vi "LocalOrGlobalMeasurement.vi"(6 "Use Offsets":T1, 7 "Tag":string, 8 "Combined":bool, 9 "IsCommand":bool, 11 "Target":T2) -> (3 "Adjusted Target":T2)   [LabVIEW 2013]
uses:
  MixedMode/Messages/Target.ctl
  Data Access Objects/Metadata/LBCB Number.ctl
  Apps/On Off Button.ctl
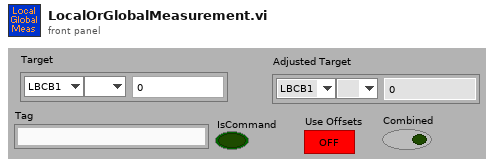
[diagram p1: front panel]
types:
  T1 = typedef "On Off Button.ctl" = bool
  T2 = typedef "Target.ctl" = cluster{"LBCB Number":T3, "DOF Vectors":enum16{" ", "Dx", "Dy", "Dz", "Rx", "Ry", "Rz", "Fx", "Fy", "Fz", "Mx", "My", "Mz"}, "Amount":dbl}
  T3 = typedef "LBCB Number.ctl" = enum16{"LBCB1", "LBCB2"}
  T4 = enum16{" ", "Dx", "Dy", "Dz", "Rx", "Ry", "Rz", "Fx", "Fy", "Fz", "Mx", "My", "Mz"}
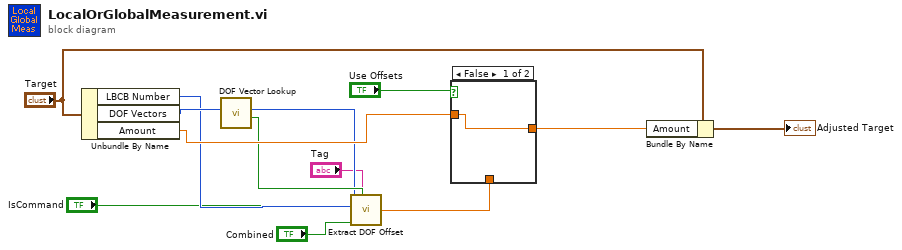
[diagram p0: block diagram]
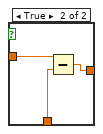
[diagram p2: hidden frame]
diagram:
  n1 = Unbundle By Name("Target") -> ("LBCB Number"=w7:T3, "DOF Vectors"=w13:T4, "Amount"=w9:dbl)
  n2 = call "DOF Vector Lookup.vi"("DOF Vectors"=w13) -> ("IsForce"=w6:bool, "Index"=w5:u32)  [unwired: 9 out]
  n3 = call "Extract DOF Offset.vi"("Tag"="Tag", "IsForce"=w6, "Combined"="Combined", "IsCommand"="IsCommand", "LBCB Number"=w7, "Index"=w5) -> ("DOF Value"=w4:dbl)
  n4 = case shown="False" "Use Offsets" {
    tunnel: w9 -> [w14 w17]
    tunnel: w4 -> [_ w16]
    tunnel: [w14 w15] -> w8
    frame False {
    }
    frame True {
      n5 = Subtract(x=w17, y=w16) -> (x-y=w15:dbl)
    }
  }
  n6 = Bundle By Name(cluster="Target", "Amount"=w8) -> (→"Adjusted Target":T2)
